vi "CleanUp.vi"(8 "Error In":errorcluster, 11 "Object in":refnum<class "Fruit.lvclass">) -> (0 "Error Out":errorcluster, 3 "object out":refnum<class "Fruit.lvclass">)   [LabVIEW 2021, in "Fruit.lvclass"]
uses:
  Fruit.lvclass
  GameEl_class/GameEl.lvclass
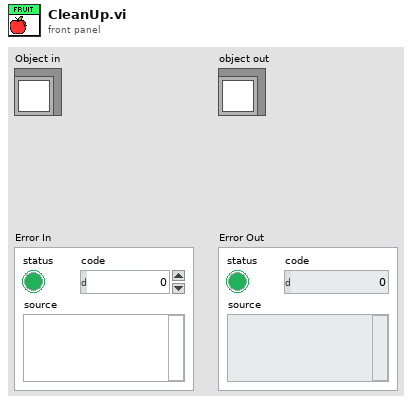
[diagram p1: front panel]
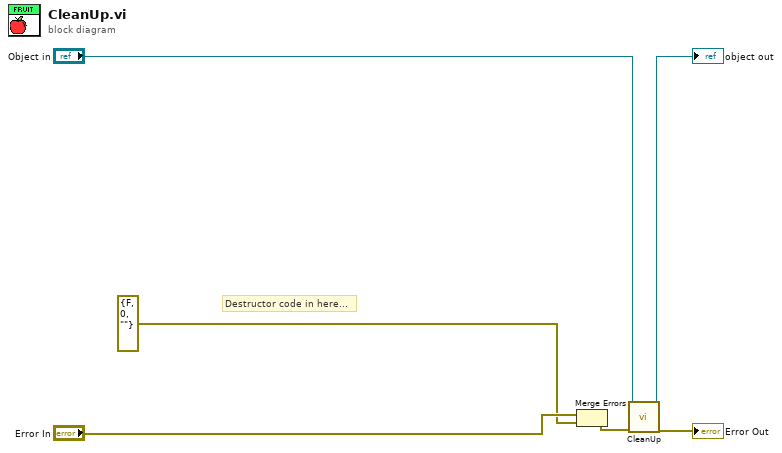
[diagram p0: block diagram]
diagram:
  # "Destructor code in here..."
  n1 = Merge Errors("Error In", errorcluster {"status"=FALSE, "code"=0, "source"=""} ("error in (no error)")) -> (w2:errorcluster)
  n2 = call-parent "CleanUp.vi"("Error In"=w2, "object in"="Object in") -> ("Error Out"=→"Error Out":errorcluster, "object out"=→"object out":refnum<class "Fruit.lvclass">)  [unwired: 8 in]
